vi "authentication.vi"(2 "Action":T2, 8 "error in (no error)":errorcluster, 9 "NewPassword":string, 10 "UserLogin":string, 11 "UserPassword":string) -> (0 "error out":errorcluster, 1 "OperationStatus":bool, 3 "Array":T1[](array[typedef]))   [LabVIEW 2024]
doc: "Auth app"
uses:
  typedefs/authentication-actions.ctl
  typedefs/account.ctl
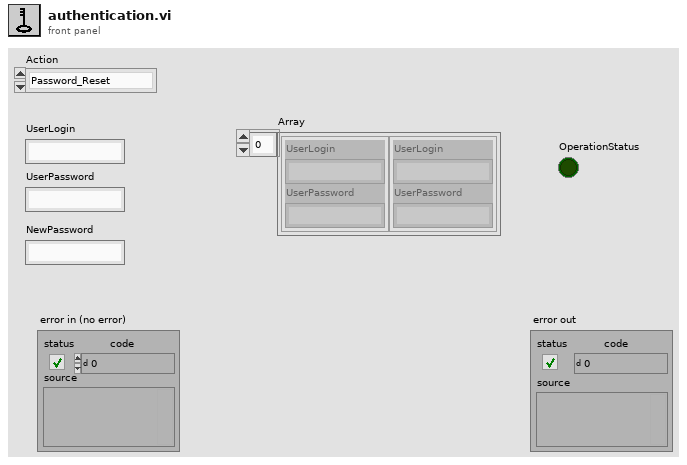
[diagram p1: front panel]
types:
  T1 = typedef "account.ctl" = cluster{"UserLogin":string, "UserPassword":string}
  T2 = typedef "authentication-actions.ctl" = enum16{"Password_Reset", "Authentication ", "Remove_Account ", "Add_Account"}
  T3 = cluster{"UserLogin":string, "UserPassword":string}
  T4 = cluster{"UserLogin":string, "UserPassword":string}[]
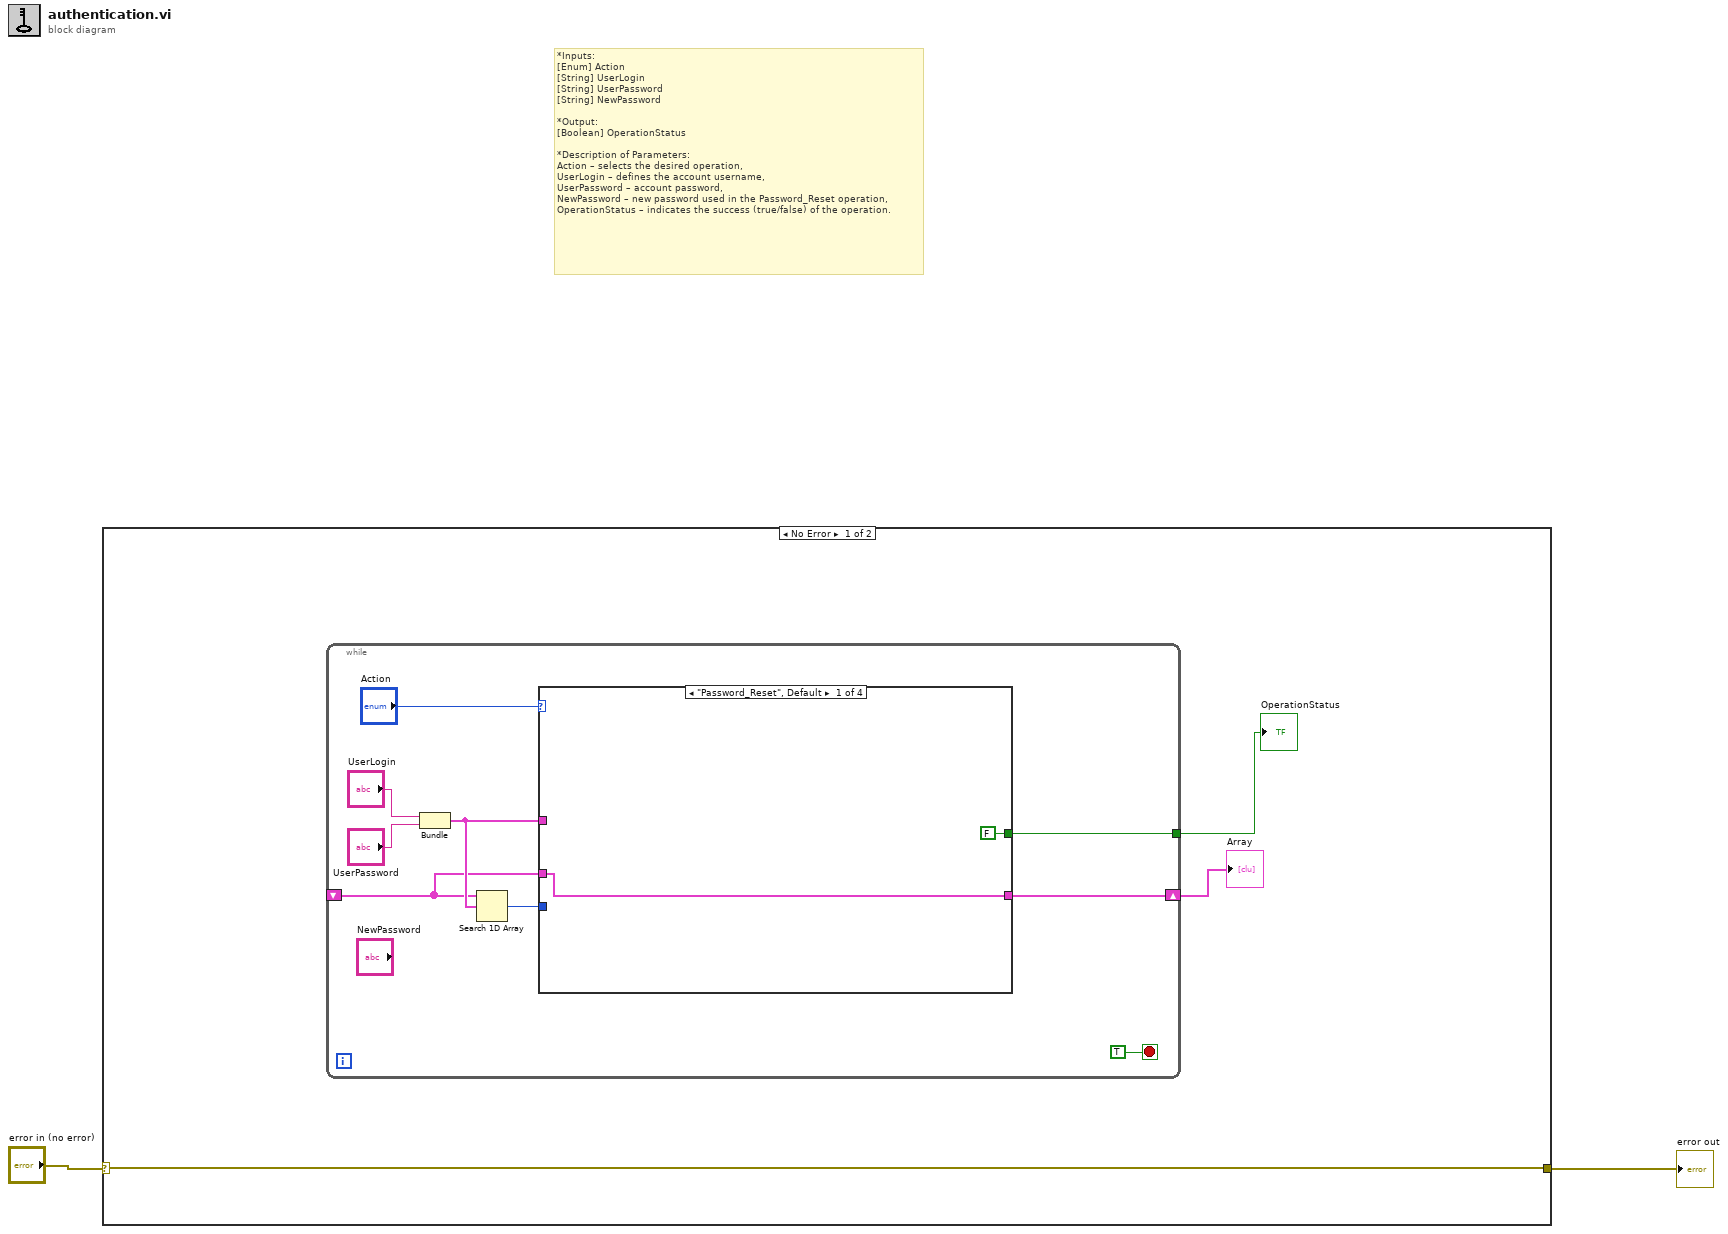
[diagram p0: block diagram]
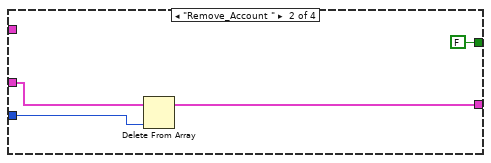
[diagram p2: hidden frame]
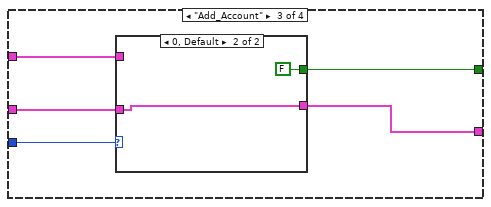
[diagram p3: hidden frame]
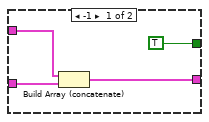
[diagram p4: hidden frame]
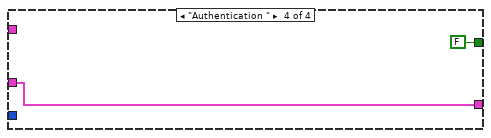
[diagram p5: hidden frame]
diagram:
  # "*Inputs:\n[Enum] Action\n[String] UserLogin\n[String] UserPassword\n[String] NewPassword\n\n*Output:\n[Boolean] OperationStatus\n\n*Description of Parameters:\nAction – selects the desired operation,\nUserLogin – defines the account username,\nUserPassword – account password,\nNewPassword – new password used in the Password_Reset operation,\nOperationStatus – indicates the success (true/false) of the operation."
  n1 = case shown="No Error" "error in (no error)" {
    selector: "error in (no error)" -> [w5 w34]
    tunnel: [w5 w34] -> w1
    frame No Error {
      n2 = while {
        shift-right: [w8] -> w4
        shift-left: _ -> [w7]
        tunnel: [w6] -> w3
        stop <- TRUE stop-if-true
        n3 = Bundle("UserLogin"="UserLogin", "UserPassword"="UserPassword") -> (w9:T3)  [unwired: 1 in]
        n4 = Search 1D Array(1D array=w7, element=w9) -> (index of element=w12:i32)  [unwired: 1 in]
        n5 = case shown="\"Password_Reset\", Default" "Action" {
          tunnel: w12 -> [_ w19 w25 _]
          tunnel: w9 -> [_ _ w24 _]
          tunnel: [w16 w18 w23 w33] -> w8
          tunnel: w7 -> [w16 w20 w22 w33]
          tunnel: [FALSE ("OperationStatus") FALSE ("OperationStatus") w21 FALSE ("OperationStatus")] -> w6
          frame "Password_Reset", Default {
          }
          frame "Remove_Account " {
            n6 = Delete From Array(array=w20, index=w19) -> (array with subset deleted=w18:T4)  [unwired: 1 in, 1 out]
          }
          frame "Add_Account" {
            n7 = case shown="0, Default" w25 {
              tunnel: w24 -> [w29 _]
              tunnel: [w28 w31] -> w23
              tunnel: w22 -> [w27 w31]
              tunnel: [TRUE ("OperationStatus") FALSE ("OperationStatus")] -> w21
              frame -1 {
                n8 = Build Array (concatenate)(w29, w27) -> (w28:T4)
              }
              frame 0, Default {
              }
            }
          }
          frame "Authentication " {
          }
        }
      }
      "OperationStatus" <- w3
      "Array" <- w4
    }
    frame Error {
    }
  }
  "error out" <- w1
